vi "Check Endpoint.vi"(8 "error in (no error)":errorcluster, 11 "Network Stream Writer in":refnum<class "Network Stream Writer.lvclass">) -> (0 "error out":errorcluster, 3 "Network Stream Writer out":refnum<class "Network Stream Writer.lvclass">)   [LabVIEW 2014, in "Network Stream Writer.lvlib" / "Network Stream Writer.lvclass"]
uses:
  Network Stream Writer.lvclass
  Network Stream Writer.lvclass/Network Stream Writer.ctl
  <resource>/objmgr/ni.dex.rc
panel:
  out "URL":string
  out "Endpoint Name":string
  out "error out 2":errorcluster
  out "Is Connected":bool
  out "Remote Endpoint Destroyed":bool
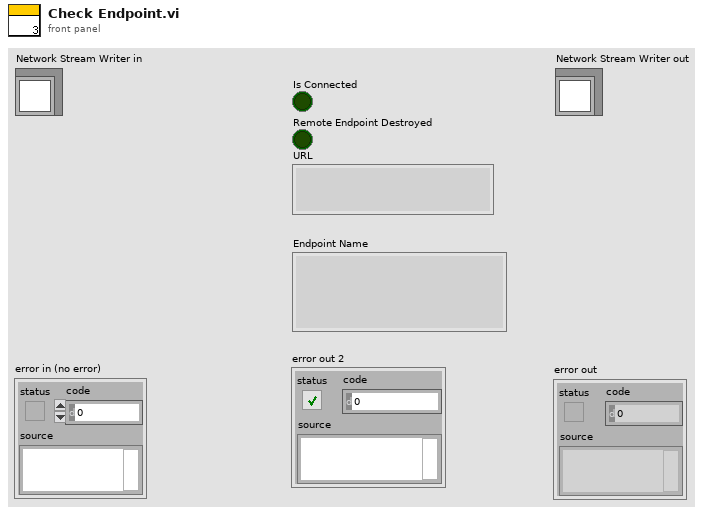
[diagram p1: front panel]
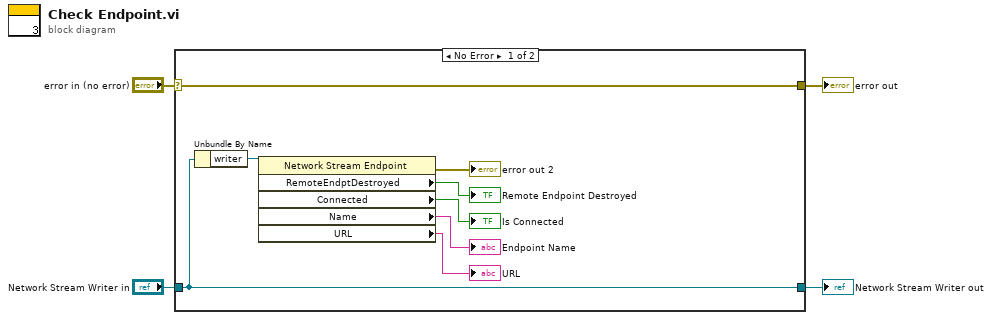
[diagram p0: block diagram]
diagram:
  n1 = case shown="No Error" "error in (no error)" {
    selector: "error in (no error)" -> [w12 w14]
    tunnel: [w12 w14] -> w3
    tunnel: [w11 w13] -> w1
    tunnel: "Network Stream Writer in" -> [w11 w13]
    frame No Error {
      n2 = Unbundle By Name(w11) -> ("writer"=w10:refnum<k21>)
      n3 = property class="Network Stream Endpoint"(reference=w10) -> (error out=→"error out 2":errorcluster, "RemoteEndptDestroyed"=→"Remote Endpoint Destroyed":bool, "Connected"=→"Is Connected":bool, "Name"=→"Endpoint Name":string, "URL"=→"URL":string)  [unwired: 1 in, 1 out]
    }
    frame Error {
    }
  }
  "error out" <- w3
  "Network Stream Writer out" <- w1
